vi "sendInt32.vi"() -> ()   [LabVIEW 2018, in "LV2Julia_core.lvlib"]
uses:
  LV2Julia_core.lvlib
  Commands.ctl
  example server response cluster.ctl
  commands LV2Jl.ctl
  cb7a600e-1a3f-45a0-9149-1773accb9ab7.vi
  Server or client state.ctl
  Julia functions enum.ctl
  c1ad7611-f00e-47ba-b950-502655f00f75.vi
  131ce374-9601-4316-a426-5169ad24f463.vi
  c49a53f7-dacd-4aad-9c2e-667c4b60ae7c.vi
  db9f0d2c-71d3-408d-98d4-5a2c4a39b6c4.vi
  <vilib>/addons/zeromq/zmq_socket.lvclass
  example args cluster.ctl
panel:
  out "parsed response 2":cluster{"elem":dbl}
  out "binary data":u8[](array[numeric])
  in  "separate arg2":cluster{"arg2":dbl}={"arg2"=2.14}
  in  "separate arg 1":cluster{"arg1":i32}={"arg1"=2}
  out "element":sgl
  in  "index to return":cluster{"idx":u16[]}={"idx"=[1, 1, 1]} {"idx" min=1}
  out "appended array":sgl[][][](array[numeric])
  in  "stop LV only":bool
  out "JSON args":string
  out "LV Client state out":T1
  out "Jl Server state out":T1
  out "size(s)":i32
  out "unsigned byte array":u8[](array[numeric])
  out "short err code":u8
  in  "go once":bool
  out "JSON received":string
  out "parsed response":T2 {"bin_lng" format="%.0e"}
  out "final error":errorcluster
  out "current error":errorcluster
  out "status":string
  in  "stop":bool
  in  "joint args":T3={"arg1"=1, "arg2"=3.14}
  in  "fun2call":T4
  # "(myf2)"
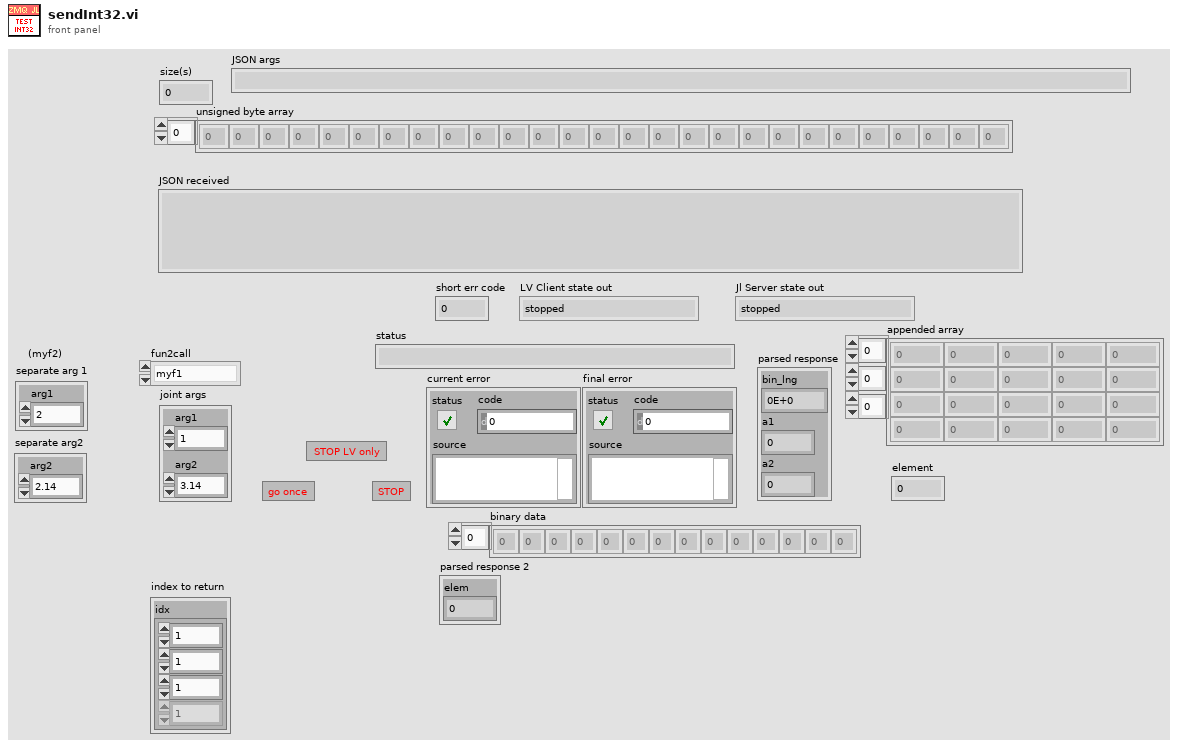
[diagram p1: front panel]
types:
  T1 = typedef "LV-0mq-Julia_roundtrip-lib.lvlib/Server or client state.ctl" = enum16{"stopped", "running", "unknown"}
  T2 = typedef "LV-0mq-Julia_roundtrip-lib.lvlib/example server response cluster.ctl" = cluster{"bin_lng":i32, "a1":i32, "a2":dbl}
  T3 = typedef "LV-0mq-Julia_roundtrip-lib.lvlib/example args cluster.ctl" = cluster{"arg1":i32, "arg2":dbl}
  T4 = typedef "Julia functions enum.ctl" = enum16{"myf1", "myf2", "myf3", "test_bin2nums", "test_rgbimg", "numarr_loopback", "numarrs_lpbk", "Not_a_Fun"}
  T5 = typedef "LV-0mq-Julia_roundtrip-lib.lvlib/Commands.ctl" = enum16{"Start Jl-server & Init LV-client", "Send request & Get response ", "Stop Jl-server & Cleanup LV-client", "Cleanup LV-client", "Start Jl-server", "Stop Jl-server", "Init LV-Client", "Cleanup LV-Client", "(not allowed)", "Set LV Client state", "Set Jl Server state", "set ZMQ timeout", "read ZMQ timeout", "read-out state"}
  T6 = typedef "LV-0mq-Julia_roundtrip-lib.lvlib/commands LV2Jl.ctl" = u8
  T7 = typedef "Bindata&description.ctl" = cluster{"bindata_descr":T8[], "bindata":u8[]}
  T8 = typedef "LV-Julia_ZMQ-Roundtrip_lib.lvlib/Bindata description.ctl" = cluster{"nofbytes":i32, "numtype":string, "start":i32, "arrdims":i32[], "kwarg_name":string, "category":string}
  T9 = typedef "LV-0mq-Julia_roundtrip-lib.lvlib/detailed error info.ctl" = cluster{"exception_or_info":string, "trace":T10[]}
  T10 = typedef "LV-0mq-Julia_roundtrip-lib.lvlib/StackFrame.ctl" = cluster{"frame_summary":string, "func":string, "linfo":string, "file":string, "line":i32, "pointer":u64, "from_c":bool, "inlined":bool}
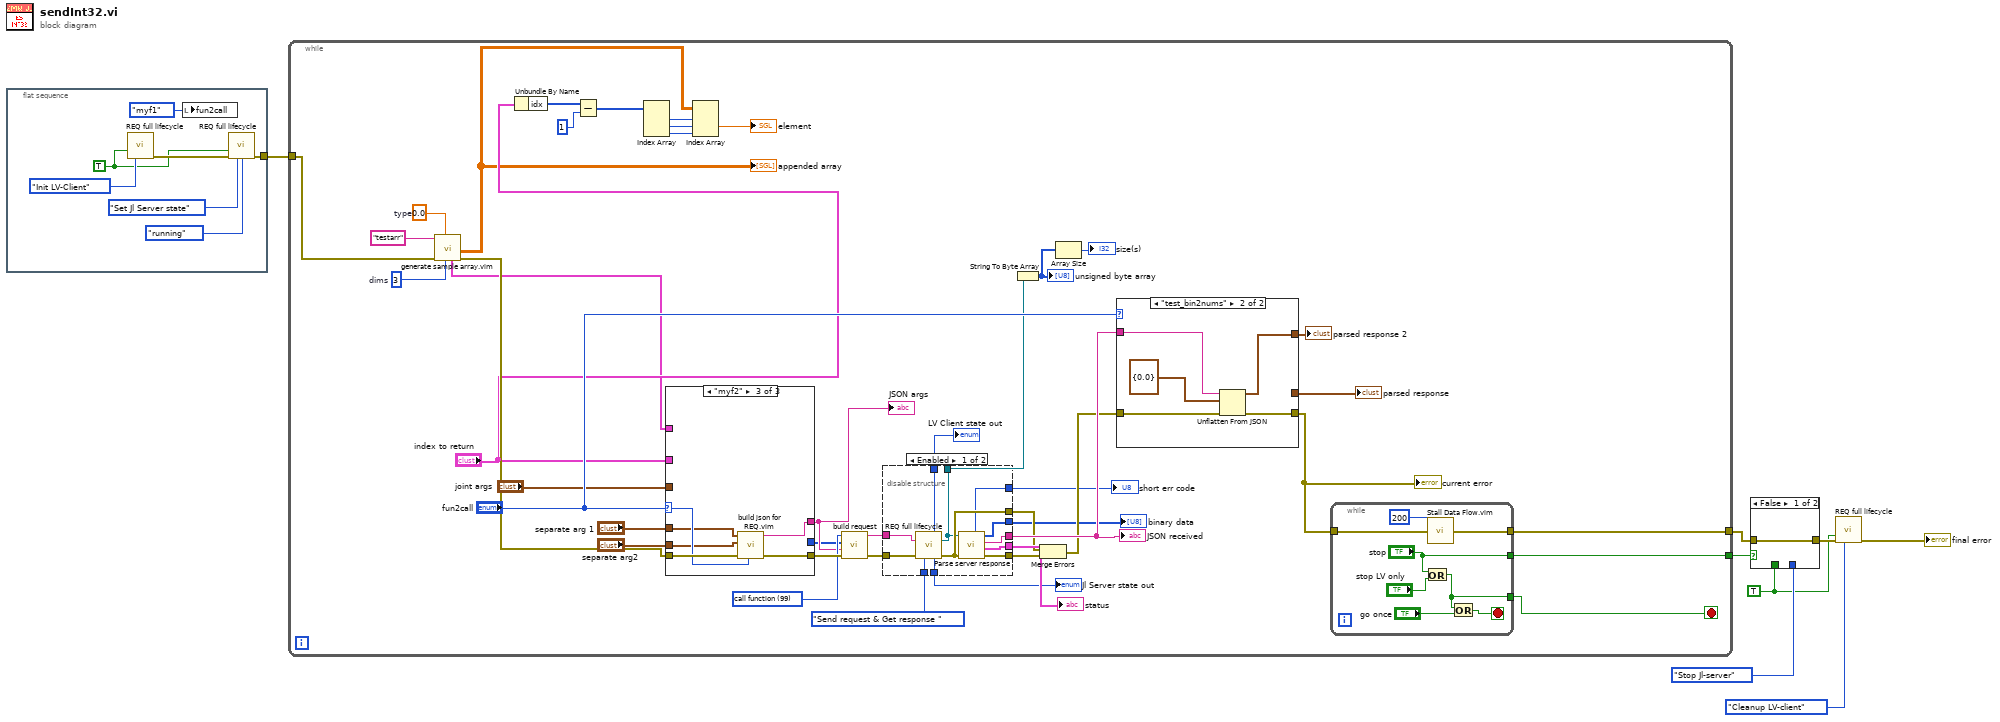
[diagram p0: block diagram]
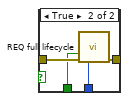
[diagram p2: hidden frame]
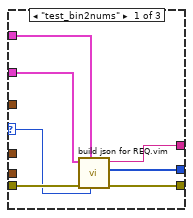
[diagram p4: hidden frame]
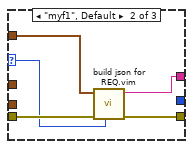
[diagram p5: hidden frame]
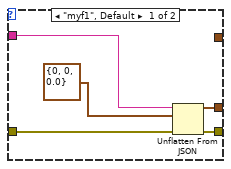
[diagram p6: hidden frame]
diagram:
  w3 = TRUE ("Force command")
  n1 = flat-sequence {
    tunnel: [w13] -> w2
    frame #0 {
      w11 = TRUE ("Force command")
      n2 = call "REQ full lifecycle.vi"("Force command"=w11, "command"=Commands."Init LV-Client") -> ("error out"=w14:errorcluster)  [unwired: 7 in, 6 out]
      n3 = local write "fun2call"(Julia_functions_enum."myf1" ("fun2call")) -> ()
      n4 = call "REQ full lifecycle.vi"("Force command"=w11, "error in"=w14, "command"=Commands."Set Jl Server state", "Jl Server state in"=Server_or_client_state."running") -> ("error out"=w13:errorcluster)  [unwired: 5 in, 6 out]
    }
  }
  n5 = while {
    tunnel: w2 -> [w35]
    tunnel: [w49] -> w8
    tunnel: [w34] -> w1
    stop <- w48 stop-if-true
    w16 = u8 3  # dims
    w18 = sgl 0.0  # type
    w46 = T6 99 items=["call function"=99, "ping"=112, "stop"=115] ("Command")
    n6 = call "generate sample array.vim"("Bindata & descr in"=w16, "type"=w18, "error in (no error)"=w35, "kwarg_name"="testarr" ("Tag")) -> ("error out"=w43:errorcluster, "Array 3D"=w17:sgl[][][], "Bindata & descr out"=w19:T7)  [unwired: 2 in, 3 out]
    "appended array" <- w17
    n7 = Unbundle By Name("index to return") -> ("idx"=w32:u16[])
    n8 = Subtract(x=w32, y=1) -> (x-y=w30:i32[])
    n9 = Index Array(array=w30) -> (element #1=w29:i32, element #2=w28:i32, element #3=w27:i32)  [unwired: 3 in]
    n10 = case shown="\"myf2\"" "fun2call" {
      selector: "fun2call" -> [w74 w79 w86]
      tunnel: [w77 w82 w88] -> w56
      tunnel: [w76 w81 w87] -> w33
      tunnel: w43 -> [w78 w83 w89]
      tunnel: w19 -> [w72 _ _]
      tunnel: "joint args" -> [_ w80 _]
      tunnel: "index to return" -> [w75 _ _]
      tunnel: [w73 _ _] -> w25
      tunnel: "separate arg 1" -> [_ _ w85]
      tunnel: "separate arg2" -> [_ _ w84]
      frame "test_bin2nums" {
        n11 = call "build json for REQ.vim"("fun2call"=w74, "Bindata & descr in"=w72, "error in (no error)"=w78, "Arguments 1"=w75) -> ("error out"=w77:errorcluster, "bindata out"=w73:u8[], "JSON string out"=w76:string)  [unwired: 5 in]
      }
      frame "myf1", Default {
        n12 = call "build json for REQ.vim"("fun2call"=w79, "error in (no error)"=w83, "Arguments 1"=w80) -> ("error out"=w82:errorcluster, "JSON string out"=w81:string)  [unwired: 6 in, 1 out]
      }
      frame "myf2" {
        n13 = call "build json for REQ.vim"("fun2call"=w86, "error in (no error)"=w89, "Arguments 2"=w84, "Arguments 1"=w85) -> ("error out"=w88:errorcluster, "JSON string out"=w87:string)  [unwired: 5 in, 1 out]
      }
    }
    "JSON args" <- w33
    n14 = Index Array(array=w17, index (dim 0)=w29, index (dim 1)=w28, index (dim 2)=w27) -> (element=→"element":sgl)
    n15 = call "build request.vi"("error in (no error)"=w56, "JSON data"=w33, "binary data"=w25, "Command"=w46) -> ("error out"=w54:errorcluster, "REQ string"=w55:string)  [unwired: 6 in]
    n16 = disable-structure shown="Enabled" {
      disable-tunnel: [w71 _] -> w59
      disable-tunnel: [w70 _] -> w58
      disable-tunnel: w55 -> [w69 _]
      disable-tunnel: w54 -> [w68 _]
      disable-tunnel: [w67 _] -> w53
      disable-tunnel: [w66 _] -> w52
      disable-tunnel: Commands."Send request & Get response " ("command") -> [w65 _]
      disable-tunnel: [w64 _] -> w41
      disable-tunnel: [w63 _] -> w40
      disable-tunnel: [w62 _] -> w37
      disable-tunnel: [w61 _] -> w36
      disable-tunnel: [w60 _] -> w22
      frame Enabled {
        n17 = call "REQ full lifecycle.vi"("data to send"=w69, "error in"=w68, "command"=w65) -> ("LV Client state out"=w61:T1, "socket out"=w63:refnum<class "zmq_socket.lvclass">, "Jl Server state out"=w62:T1, "error out"=w66:errorcluster)  [unwired: 6 in, 3 out]
        n18 = call "Parse server response.vi"("error in (no error)"=w66, "server response in"=w63) -> ("error out"=w67:errorcluster, "detailed error info"=w71:T9, "JSON out"=w70:string, "binary data"=w60:u8[], "return code"=w64:u8)  [unwired: 2 in, 3 out]
      }
      frame Disabled {
      }
    }
    "status" <- w59
    "JSON received" <- w58
    "short err code" <- w41
    "Jl Server state out" <- w37
    "LV Client state out" <- w36
    "binary data" <- w22
    n19 = String To Byte Array(string=w40) -> (unsigned byte array=w39:u8[])
    "unsigned byte array" <- w39
    n20 = Merge Errors(w52, w53) -> (w57:errorcluster)
    n21 = Array Size(array=w39) -> (size(s)=→"size(s)":i32)
    n22 = case shown="\"test_bin2nums\"" "fun2call" {
      tunnel: w58 -> [w102 w107]
      tunnel: w57 -> [w101 w106]
      tunnel: [w100 w105] -> w50
      tunnel: [w99 _] -> w47
      tunnel: [_ w103] -> w21
      frame "myf1", Default {
        n23 = Unflatten From JSON(JSON string=w102, type and defaults=T2 {"bin_lng"=0, "a1"=0, "a2"=0.0} ("parsed response"), error in (no error)=w101) -> (value=w99:T2, error out=w100:errorcluster)  [unwired: 4 in]
      }
      frame "test_bin2nums" {
        n24 = Unflatten From JSON(JSON string=w107, type and defaults=cluster{"elem":dbl} {"elem"=0.0} ("parsed response"), error in (no error)=w106) -> (value=w103:cluster{"elem":dbl}, error out=w105:errorcluster)  [unwired: 4 in]
      }
    }
    "current error" <- w50
    "parsed response" <- w47
    "parsed response 2" <- w21
    n25 = while {
      tunnel: w50 -> [w97]
      tunnel: [w96] -> w49
      tunnel: [w92] -> w48
      tunnel: ["stop"] -> w34
      stop <- w93 stop-if-true
      n26 = Or(x="stop", y="stop LV only") -> (x .or. y?=w92:bool)
      n27 = call "Stall Data Flow.vim"("value in"=w97, "milliseconds to wait"=u32 200) -> ("value out"=w96:errorcluster)  [unwired: 1 out]
      n28 = Or(x=w92, y="go once") -> (x .or. y?=w93:bool)
    }
  }
  n29 = case shown="False" w1 {
    tunnel: w8 -> [w108 w112]
    tunnel: Commands."Stop Jl-server" ("command") -> [_ w111]
    tunnel: [w108 w110] -> w6
    tunnel: w3 -> [_ w109]
    frame False {
    }
    frame True {
      n30 = call "REQ full lifecycle.vi"("Force command"=w109, "error in"=w112, "command"=w111) -> ("error out"=w110:errorcluster)  [unwired: 6 in, 6 out]
    }
  }
  n31 = call "REQ full lifecycle.vi"("Force command"=w3, "error in"=w6, "command"=Commands."Cleanup LV-client") -> ("error out"=→"final error":errorcluster)  [unwired: 6 in, 6 out]
